vi "FindVISAResource.vi"() -> ()   [LabVIEW 2014]
uses:
  <vilib>/Instr/_visa.llb/VISA Find Search Mode.ctl
  <vilib>/Instr/_visa.llb/VISA Configure Serial Port (Instr).vi
panel:
  out "error out":errorcluster
  out "OUT COM":refnum<visa-resource-name>
  in  "baud rate (9600)":u32=9600
  out "find list":string[](array[string])
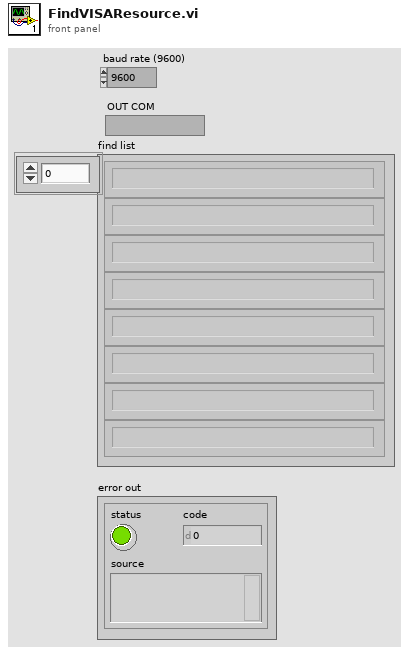
[diagram p1: front panel]
types:
  T1 = typedef "VISA Find Search Mode.ctl" = u32
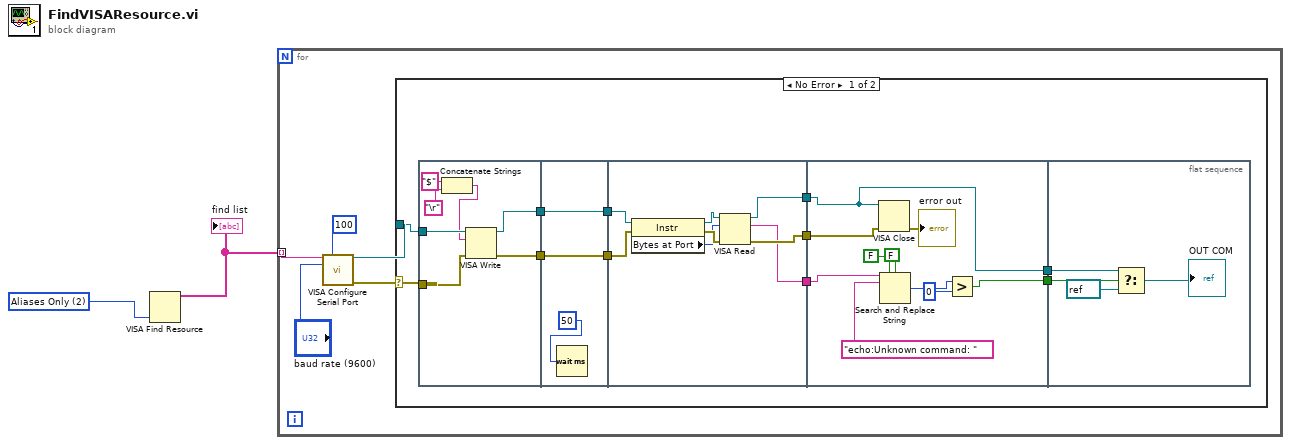
[diagram p0: block diagram]
diagram:
  w2 = T1 2 items=["Canonical Names Only"=0, "Aliases Only"=2, "Include Matching Aliases"=3, "Include All Aliases"=4] ("Search Mode")
  n1 = VISA Find Resource(10:w2) -> (3:w1:string[])  [unwired: 2 in, 2 out]
  "find list" <- w1
  n2 = for {
    tunnel: w1 -> [w7] mode=indexing
    n3 = call-poly "VISA Configure Serial Port"("VISA resource name"=w7, "timeout (10sec)"=u32 100, "baud rate (9600)"="baud rate (9600)") -> ("VISA resource name out"=w4:refnum<visa-resource-name>, "error out"=w5:errorcluster)  [unwired: 11 in]
    n4 = case shown="No Error" w5 {
      selector: w5 -> [w13 _]
      tunnel: w4 -> [w14 _]
      frame No Error {
        n5 = flat-sequence {
          tunnel: [w24] -> w18
          tunnel: [w23] -> w17
          tunnel: w14 -> [w25]
          tunnel: w13 -> [w19]
          tunnel: [w27] -> w16
          tunnel: w18 -> [w27]
          tunnel: w17 -> [w26]
          tunnel: [w26] -> w15
          tunnel: w16 -> [w34]
          tunnel: w15 -> [w33]
          tunnel: [w36] -> w12
          tunnel: [w35] -> w11
          tunnel: [w29] -> w10
          tunnel: w12 -> [w43]
          tunnel: w11 -> [w42]
          tunnel: w10 -> [w38]
          tunnel: [w39] -> w9
          tunnel: [w38] -> w8
          tunnel: w9 -> [w50]
          tunnel: w8 -> [w49]
          frame #0 {
            n6 = Concatenate Strings("$" ("string"), "\r") -> (w20:string)
            n7 = VISA Write(VISA resource name=w25, write buffer=w20, error in (no error)=w19) -> (VISA resource name out=w24:refnum<visa-resource-name>, error out=w23:errorcluster)  [unwired: 1 out]
          }
          frame #1 {
            n8 = Wait (ms)(milliseconds to wait=u32 50 ("millisecond timer value")) -> ()  [unwired: 1 out]
          }
          frame #2 {
            n9 = property class="Instr"(reference=w34, error in=w33) -> (reference out=w32:refnum<visa-resource-name>, error out=w31:errorcluster, "Bytes at Port"=w30:u32)
            n10 = VISA Read(VISA resource name=w32, byte count=w30, error in (no error)=w31) -> (VISA resource name out=w29:refnum<visa-resource-name>, read buffer=w35:string, error out=w36:errorcluster)  [unwired: 1 out]
          }
          frame #3 {
            n11 = VISA Close(VISA resource name=w38, error in (no error)=w43) -> (error out=→"error out":errorcluster)
            n12 = Search and Replace String(replace all?=FALSE ("replace all? (F)"), case sensitive?=FALSE ("ignore case? (F)"), input string=w42, search string="echo:Unknown command: ") -> (number of replacements=w41:i32)  [unwired: 4 in, 3 out]
            n13 = Greater?(x=w41, y=0) -> (0:w39:bool)
          }
          frame #4 {
            n14 = Select(t=w49, s=w50, f=refnum<visa-resource-name> refnum) -> (s? t:f=→"OUT COM":refnum<visa-resource-name>)
          }
        }
      }
      frame Error {
      }
    }
  }
